vi "DiagnosticsCameratest.vi"() -> ()   [LabVIEW 2010]
panel:
  out "PvCam Minor Version":u32
  out "Major Version":u32
  out "PCI FW Ver":u32
  out "Camera FW ver":u32
  out "Camera Serial Num":u32
  out "PvCam Trivial Ver":u32
  out "Device Driver Ver":u32
  out "Internal Build":u32
  out "External Build":u32
  out "Minor Version":u32
  out "Major Version":u32
  out "Total Number of Devices":u32
  out "error out":errorcluster
  in  "error in (no error)":errorcluster
  # "Low Level Driver Version"
  # "Toolkit Version"
  # "DiagnosticsCameraTest:\n\n1.) Make sure the camera is turned on and connected."
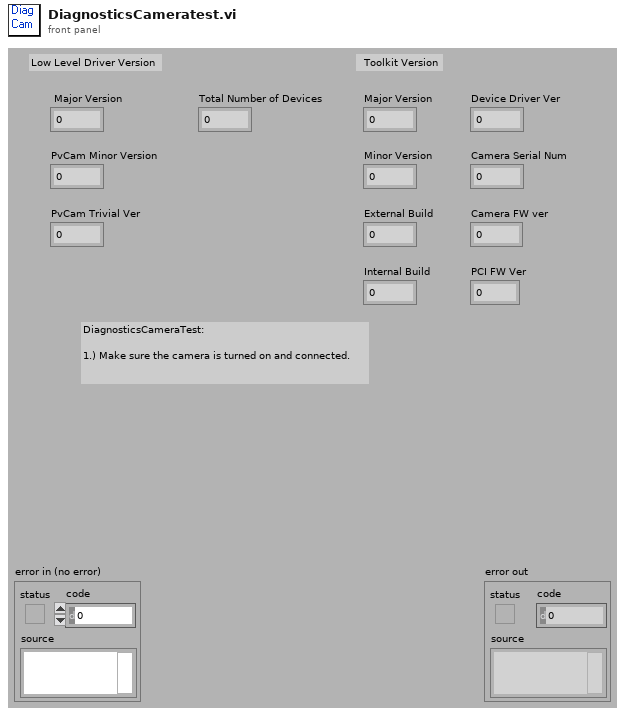
[diagram p1: front panel]
types:
  T1 = cluster{"Major Version":u32, "Minor Version":u32, "External Build":u32, "Internal Build":u32}
  T2 = cluster{"PvCam DLL Ver":u32, "Camera Serial Number ":u32, "Device Driver Ver":u32, "Camera FW Ver":u32, "PCI FW Ver":u32}
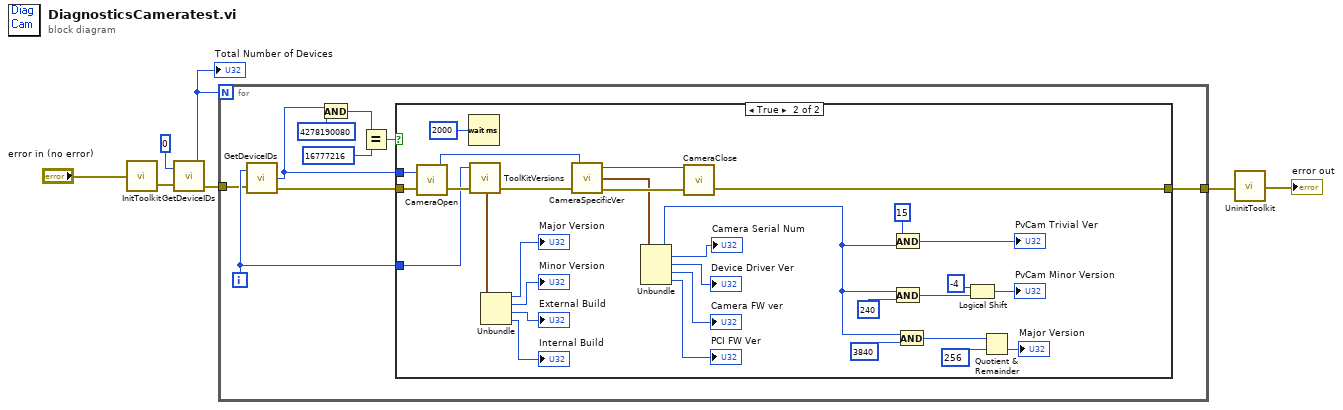
[diagram p0: block diagram]
diagram:
  n1 = call <userlib>:"InitToolkit.vi"("error in"="error in (no error)") -> ("error out"=w6:errorcluster)
  n2 = call <userlib>:"GetDeviceIDs.vi"("Index"=u32 0, "error in"=w6) -> ("Total Nuber of Devices or DLLs"=w4:u32, "error out"=w3:errorcluster)  [unwired: 1 out]
  "Total Number of Devices" <- w4
  n3 = for {
    N: w4 -> [_]
    tunnel: [w14] -> w2
    tunnel: w3 -> [w12]
    i -> [w16]
    n4 = call <userlib>:"GetDeviceIDs.vi"("Index"=w16, "error in"=w12) -> ("Device ID"=w10:u32, "error out"=w11:errorcluster)  [unwired: 1 out]
    n5 = And(x=w10, y=u32 4278190080) -> (x .and. y?=w9:u32)
    n6 = Equal?(x=w9, y=u32 16777216) -> (x = y?=w13:bool)
    n7 = case shown="True" w13 {
      tunnel: w16 -> [_ w36]
      tunnel: w11 -> [w17 w33]
      tunnel: [w17 w48] -> w14
      tunnel: w10 -> [_ w32]
      frame False {
      }
      frame True {
        n8 = call <userlib>:"CameraOpen.vi"("error in"=w33, "Camera Device ID"=w32) -> ("error out"=w37:errorcluster, "Camera Handle"=w35:u32)
        n9 = Wait (ms)(milliseconds to wait=u32 2000) -> ()  [unwired: 1 out]
        n10 = call <userlib>:"ToolKitVersions.vi"("error in"=w37, "Index"=w36) -> ("error out"=w34:errorcluster, "Versions"=w39:T1)  [unwired: 1 in, 1 out]
        n11 = Unbundle(w39) -> ("Major Version"=→"Major Version":u32, "Minor Version"=→"Minor Version":u32, "External Build"=→"External Build":u32, "Internal Build"=→"Internal Build":u32)
        n12 = call <userlib>:"CameraSpecificVer.vi"("error in (no error)"=w34, "Camera Handle"=w35) -> ("error out"=w47:errorcluster, "Camera Specific Versions"=w45:T2, "Camera Handle"=w46:u32)  [unwired: 1 in]
        n13 = Unbundle(w45) -> ("PvCam DLL Ver"=w29:u32, "Camera Serial Number"=→"Camera Serial Num":u32, "Device Driver Ver"=→"Device Driver Ver":u32, "Camera FW Ver"=→"Camera FW ver":u32, "PCI FW Ver"=→"PCI FW Ver":u32)
        n14 = call <userlib>:"CameraClose.vi"("error in"=w47, "Camera Handle"=w46) -> ("error out"=w48:errorcluster)
        n15 = And(x=u32 15, y=w29) -> (x .and. y?=→"PvCam Trivial Ver":u32)
        n16 = And(x=w29, y=u32 240) -> (x .and. y?=w19:u32)
        n17 = And(x=w29, y=u32 3840) -> (x .and. y?=w25:u32)
        n18 = Logical Shift(y=i16 -4, x=w19) -> (x << y=→"PvCam Minor Version":u32)
        n19 = Quotient & Remainder(x=w25, y=u32 256) -> (floor(x/y)=→"Major Version":u32)  [unwired: 1 out]
      }
    }
  }
  n20 = call <userlib>:"UninitToolkit.vi"("error in"=w2) -> ("error out"=→"error out":errorcluster)
